vi "Calculate_Volume.vi"(1 "Boxes Dimensions":T1[](array[typedef])) -> (0 "Sorted Boxes":T1[](array[typedef]))   [LabVIEW 2015]
uses:
  Controls/Box_Properties.ctl
  Controls/Box_Location.ctl
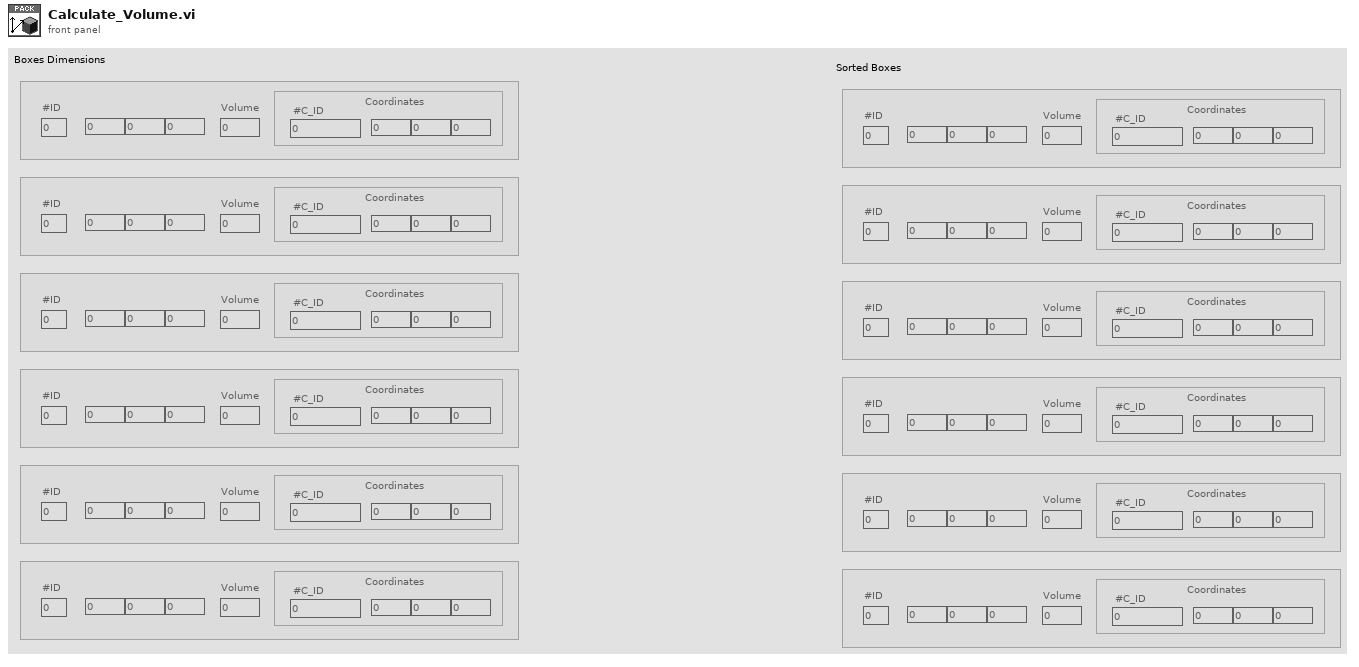
[diagram p1: front panel]
types:
  T1 = typedef "Box_Properties.ctl" = cluster{"Boxes Dimensions":dbl[], "Volume":dbl, "#ID":dbl, "Location":T2}
  T2 = typedef "Box_Location.ctl" = cluster{"#C_ID":dbl, "Coordinates":dbl[]}
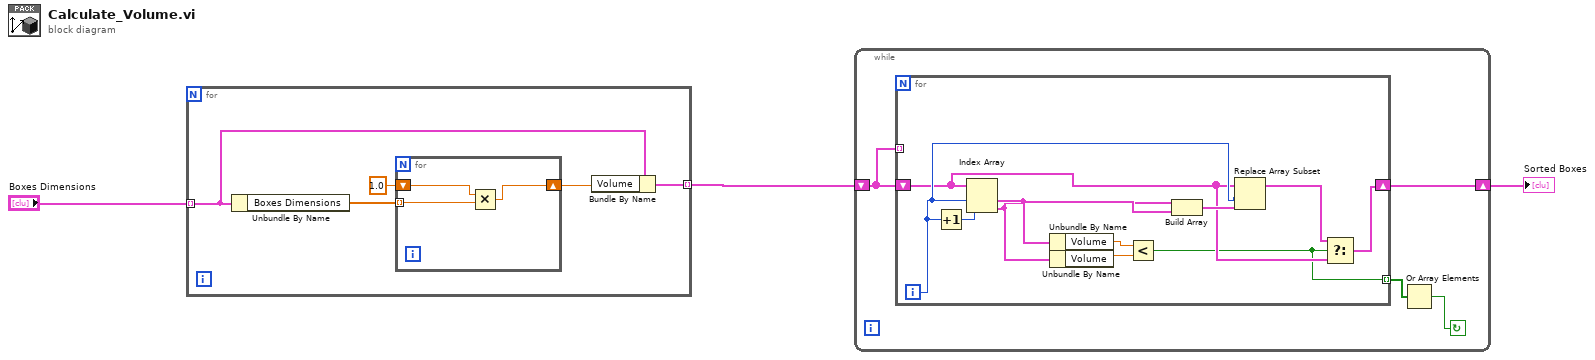
[diagram p0: block diagram]
diagram:
  n1 = for {
    tunnel: "Boxes Dimensions" -> [w6] mode=indexing
    tunnel: [w5] -> w2 mode=indexing
    n2 = Unbundle By Name(w6) -> ("Boxes Dimensions"=w8:dbl[])
    n3 = for {
      tunnel: w8 -> [w11] mode=indexing
      shift-right: [w9] -> w4
      shift-left: 1.0 -> [w10]
      n4 = Multiply(x=w10, y=w11) -> (x*y=w9:dbl)
    }
    n5 = Bundle By Name(cluster=w6, "Volume"=w4) -> (w5:T1)
  }
  n6 = while {
    shift-right: [w12] -> w1
    shift-left: w2 -> [w15]
    stop <- w14 continue-if-true
    n7 = for {
      shift-right: [w18] -> w12
      shift-left: w15 -> [w17]
      tunnel: w15 -> [_] mode=indexing
      tunnel: [w16] -> w13 mode=indexing
      i -> [w23]
      n8 = Increment(x=w23) -> (x+1=w26:i32)
      n9 = Index Array(array=w17, index #1=w23, index #2=w26) -> (element #1=w22:T1, element #2=w21:T1)
      n10 = Unbundle By Name(w22) -> ("Volume"=w25:dbl)
      n11 = Unbundle By Name(w21) -> ("Volume"=w24:dbl)
      n12 = Less?(x=w25, y=w24) -> (x < y?=w16:bool)
      n13 = Build Array(w21, w22) -> (w20:T1[])
      n14 = Replace Array Subset(array=w17, new element=w20, index=w23) -> (w19:T1[])
      n15 = Select(t=w19, s=w16, f=w17) -> (s? t:f=w18:T1[])
    }
    n16 = Or Array Elements(Boolean array=w13) -> (logical OR=w14:bool)
  }
  "Sorted Boxes" <- w1
